vi "Validate Receive Mode Codes.vi"(4 "RT Address (0-30)":u8, 6 "RT 1?":bool, 8 "error in (no error)":errorcluster, 11 "1553 Unit Test in":refnum<class "Remote Terminal.lvclass">) -> (0 "error out":errorcluster, 3 "1553 Unit Test out":refnum<class "Remote Terminal.lvclass">)   [LabVIEW 2020, in "Unit Tests.lvlib" / "Remote Terminal.lvclass"]
uses:
  Remote Terminal.lvclass
  Remote Terminal.lvclass/Remote Terminal.ctl
  <vilib>/addons/_JKI Toolkits/Caraya/classes/Assert/Assert True.vi
  Dependencies/FPGA Interface/FPGA Interface.lvclass
  <vilib>/addons/_JKI Toolkits/Caraya/classes/Assert/Assert.lvclass
  <vilib>/addons/_JKI Toolkits/Caraya/classes/Test/Test.lvclass
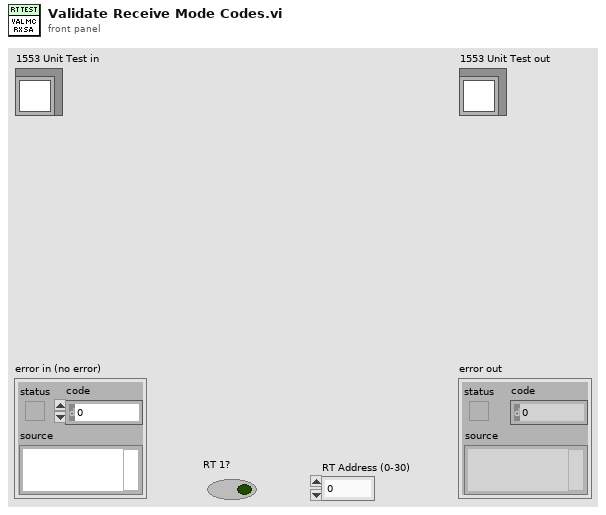
[diagram p1: front panel]
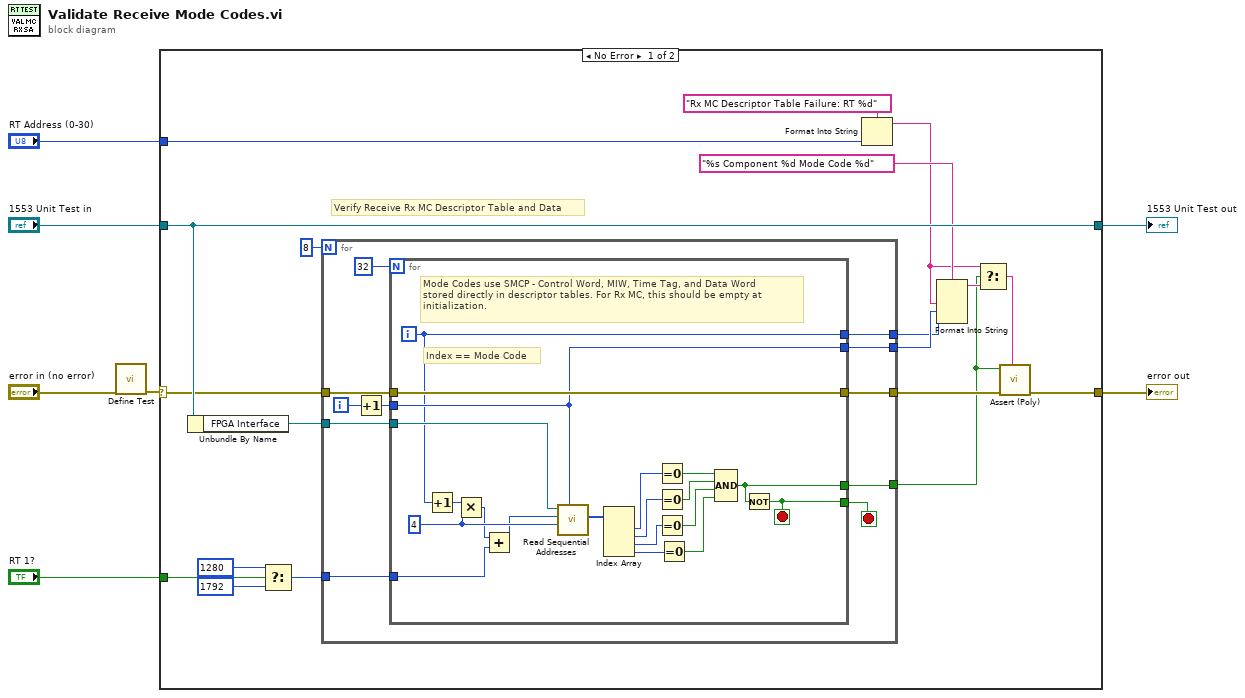
[diagram p0: block diagram]
diagram:
  n1 = call <vilib>:"Define Test.vi"("error in (no error)"="error in (no error)") -> ("error out"=w3:errorcluster)  [unwired: 9 in, 1 out]
  n2 = case shown="No Error" w3 {
    selector: w3 -> [w19 w59]
    tunnel: [w18 w59] -> w7
    tunnel: [w26 w58] -> w5
    tunnel: "1553 Unit Test in" -> [w26 w58]
    tunnel: "RT 1?" -> [w22 _]
    tunnel: "RT Address (0-30)" -> [w13 _]
    frame No Error {
      # "Verify Receive Rx MC Descriptor Table and Data"
      n3 = Unbundle By Name(w26) -> ("FPGA Interface"=w20:refnum<class "FPGA Interface.lvclass">)
      n4 = Select(t=u16 1280, s=w22, f=u16 1792) -> (s? t:f=w21:u16)
      n5 = for {
        N: 8 -> [_]
        tunnel: w21 -> [w29]
        tunnel: w20 -> [w34]
        tunnel: w19 -> [w33]
        tunnel: [w32] -> w9
        tunnel: [w31] -> w11
        tunnel: [w30] -> w10
        tunnel: [w28] -> w8
        i -> [w37]
        stop <- w27 stop-if-true
        n6 = Increment(x=w37) -> (x+1=w35:i32)
        n7 = for {
          N: 32 -> [_]
          tunnel: w35 -> [w55]
          tunnel: w34 -> [w57]
          tunnel: w33 -> [w56]
          tunnel: [w56] -> w32
          tunnel: [w40] -> w28
          tunnel: [w55] -> w31
          tunnel: [w49] -> w30
          tunnel: w29 -> [w51]
          tunnel: [w39] -> w27
          i -> [w49]
          stop <- w39 stop-if-true
          w53 = u16 4 ("x")
          # "Mode Codes use SMCP - Control Word, MIW, Time Tag, and Data Word \nstored directly in descriptor tables. For Rx MC, this should be empty at\ninitialization."
          # "Index == Mode Code"
          n8 = Increment(x=w49) -> (x+1=w38:i32)
          n9 = Multiply(x=w38, y=w53) -> (x*y=w52:i32)
          n10 = Add(x=w52, y=w51) -> (x+y=w50:i32)
          n11 = call-dynamic "Read Sequential Addresses.vi"("Target IC (1-8)"=w55, "Addresses to Read"=w53, "Starting Address"=w50, "FPGA Interface in"=w57) -> ("Data"=w54:u16[])  [unwired: 6 in, 1 out]
          n12 = Index Array(array=w54) -> (element #1=w48:u16, element #2=w47:u16, element #3=w46:u16, element #4=w45:u16)  [unwired: 4 in]
          n13 = Equal To 0?(x=w48) -> (x = 0?=w44:bool)
          n14 = Equal To 0?(x=w47) -> (x = 0?=w43:bool)
          n15 = Equal To 0?(x=w46) -> (x = 0?=w42:bool)
          n16 = Equal To 0?(x=w45) -> (x = 0?=w41:bool)
          n17 = Compound Arithmetic op=AND(w44, w43, w42, w41) -> (w40:bool)
          n18 = Not(x=w40) -> (.not. x?=w39:bool)
        }
      }
      n19 = Format Into String(format string="Rx MC Descriptor Table Failure: RT %d" ("message (\"\")"), w13) -> (resulting string=w12:string)  [unwired: 2 in, 1 out]
      n20 = Format Into String(format string="%s Component %d Mode Code %d" ("message (\"\")"), w12, w11, w10) -> (resulting string=w16:string)  [unwired: 2 in, 1 out]
      n21 = Select(t=w12, s=w8, f=w16) -> (s? t:f=w15:string)
      n22 = call-poly <vilib>:"Assert (Poly).vi"("Label"=w15, "error in (no error)"=w9, "True?"=w8) -> ("error out"=w18:errorcluster)  [unwired: 7 in, 1 out]
    }
    frame Error {
    }
  }
  "error out" <- w7
  "1553 Unit Test out" <- w5
